vi "RTS APLUS Open Close.vi"(7 "Open Connection?":bool, 8 "error in (no error)":errorcluster, 9 "Modbus Remote Port":u16, 10 "RTS Config Setup Output":T4, 11 "Modbus Connections In":T1={"Wago ModBus Connection"=refnum, "APLUS 1 Modbus Connection"=refnum, "APLUS 2 Modbus Connection"=refnum, "APLUS 3 Modbus Connection"=refnum, "APLUS 4 Modbus Connection"=refnum, "APLUS 5 Modbus Connection"=refnum, "APLUS 6 Modbus Connection"=refnum, "APLUS 7 Modbus Connection"=refnum, "APLUS 8 Modbus Connection"=refnum, "MX 1 VISA Connection"="", "MX 2 VISA Connection"="", "MX 3 VISA Connection"="", "MX 4 VISA Connection"="", "MX 5 VISA Connection"="", "MX1"={"Base Time"=0, "Session Number"=0, "Last Data Number"={"High"=-1, "Low"=4294967295}, "Channel List"=[], "FIFO Number (0)"=0, "Channel Number (1)"=1, "Select FIFO or Channel (F:Channel)"=FALSE, "MX100 Data"={"Measurement Values out"=[], "Date/Time"=""}}, "MX2"={"Base Time"=0, "Session Number"=0, "Last Data Number"={"High"=-1, "Low"=4294967295}, "Channel List"=[], "FIFO Number (0)"=0, "Channel Number (1)"=1, "Select FIFO or Channel (F:Channel)"=FALSE, "MX100 Data"={"Measurement Values out"=[], "Date/Time"=""}}, "MX3"={"Base Time"=0, "Session Number"=0, "Last Data Number"={"High"=-1, "Low"=4294967295}, "Channel List"=[], "FIFO Number (0)"=0, "Channel Number (1)"=1, "Select FIFO or Channel (F:Channel)"=FALSE, "MX100 Data"={"Measurement Values out"=[], "Date/Time"=""}}, "MX4"={"Base Time"=0, "Session Number"=0, "Last Data Number"={"High"=-1, "Low"=4294967295}, "Channel List"=[], "FIFO Number (0)"=0, "Channel Number (1)"=1, "Select FIFO or Channel (F:Channel)"=FALSE, "MX100 Data"={"Measurement Values out"=[], "Date/Time"=""}}, "MX5"={"Base Time"=0, "Session Number"=0, "Last Data Number"={"High"=-1, "Low"=4294967295}, "Channel List"=[], "FIFO Number (0)"=0, "Channel Number (1)"=1, "Select FIFO or Channel (F:Channel)"=FALSE, "MX100 Data"={"Measurement Values out"=[], "Date/Time"=""}}} {"MX5"."Channel Number (1)" min=1 max=60 step=1; "MX5"."FIFO Number (0)" min=-1 max=2 step=1; "MX4"."Channel Number (1)" min=1 max=60 step=1; "MX4"."FIFO Number (0)" min=-1 max=2 step=1; "MX3"."Channel Number (1)" min=1 max=60 step=1; "MX3"."FIFO Number (0)" min=-1 max=2 step=1; "MX2"."Channel Number (1)" min=1 max=60 step=1; "MX2"."FIFO Number (0)" min=-1 max=2 step=1; "MX1"."Channel Number (1)" min=1 max=60 step=1; "MX1"."FIFO Number (0)" min=-1 max=2 step=1}) -> (0 "error out":errorcluster, 3 "Modbus Connections Out":T1={"Wago ModBus Connection"=refnum, "APLUS 1 Modbus Connection"=refnum, "APLUS 2 Modbus Connection"=refnum, "APLUS 3 Modbus Connection"=refnum, "APLUS 4 Modbus Connection"=refnum, "APLUS 5 Modbus Connection"=refnum, "APLUS 6 Modbus Connection"=refnum, "APLUS 7 Modbus Connection"=refnum, "APLUS 8 Modbus Connection"=refnum, "MX 1 VISA Connection"="", "MX 2 VISA Connection"="", "MX 3 VISA Connection"="", "MX 4 VISA Connection"="", "MX 5 VISA Connection"="", "MX1"={"Base Time"=0, "Session Number"=0, "Last Data Number"={"High"=-1, "Low"=4294967295}, "Channel List"=[], "FIFO Number (0)"=0, "Channel Number (1)"=1, "Select FIFO or Channel (F:Channel)"=FALSE, "MX100 Data"={"Measurement Values out"=[], "Date/Time"=""}}, "MX2"={"Base Time"=0, "Session Number"=0, "Last Data Number"={"High"=-1, "Low"=4294967295}, "Channel List"=[], "FIFO Number (0)"=0, "Channel Number (1)"=1, "Select FIFO or Channel (F:Channel)"=FALSE, "MX100 Data"={"Measurement Values out"=[], "Date/Time"=""}}, "MX3"={"Base Time"=0, "Session Number"=0, "Last Data Number"={"High"=-1, "Low"=4294967295}, "Channel List"=[], "FIFO Number (0)"=0, "Channel Number (1)"=1, "Select FIFO or Channel (F:Channel)"=FALSE, "MX100 Data"={"Measurement Values out"=[], "Date/Time"=""}}, "MX4"={"Base Time"=0, "Session Number"=0, "Last Data Number"={"High"=-1, "Low"=4294967295}, "Channel List"=[], "FIFO Number (0)"=0, "Channel Number (1)"=1, "Select FIFO or Channel (F:Channel)"=FALSE, "MX100 Data"={"Measurement Values out"=[], "Date/Time"=""}}, "MX5"={"Base Time"=0, "Session Number"=0, "Last Data Number"={"High"=-1, "Low"=4294967295}, "Channel List"=[], "FIFO Number (0)"=0, "Channel Number (1)"=1, "Select FIFO or Channel (F:Channel)"=FALSE, "MX100 Data"={"Measurement Values out"=[], "Date/Time"=""}}} {"MX5"."Channel Number (1)" min=1 max=60 step=1; "MX5"."FIFO Number (0)" min=-1 max=2 step=1; "MX4"."Channel Number (1)" min=1 max=60 step=1; "MX4"."FIFO Number (0)" min=-1 max=2 step=1; "MX3"."Channel Number (1)" min=1 max=60 step=1; "MX3"."FIFO Number (0)" min=-1 max=2 step=1; "MX2"."Channel Number (1)" min=1 max=60 step=1; "MX2"."FIFO Number (0)" min=-1 max=2 step=1; "MX1"."Channel Number (1)" min=1 max=60 step=1; "MX1"."FIFO Number (0)" min=-1 max=2 step=1})   [LabVIEW 2016]
uses:
  Type Definitions/RTS Modbus Connections.ctl
  <vilib>/NI/Modbus Library/API/Master/Modbus Master.lvclass
  Drivers/Yokogawa MX100/Type Definitions/MX100 Initialization.ctl
  Drivers/Yokogawa MX100/Type Definitions/MX100 Data.ctl
  Type Definitions/RTS Configuration Setup.ctl
  Type Definitions/RTS Wago Config.ctl
  Type Definitions/RTS APLUS Config.ctl
  Type Definitions/RTS Yokogawa MX Config.ctl
  Type Definitions/RTS Replay Server Control.ctl
  Type Definitions/RTS Server Configuration.ctl
  Type Definitions/RTS Station Settions TCP Comms.ctl
  Type Definitions/RTS Chamber Save Status.ctl
  Type Definitions/RTS Test Pattern.ctl
  <vilib>/NI/Modbus Library/API/Wrapper/Create TCP Master.vi
  <vilib>/NI/Modbus Library/API/Wrapper/API Main.lvlib
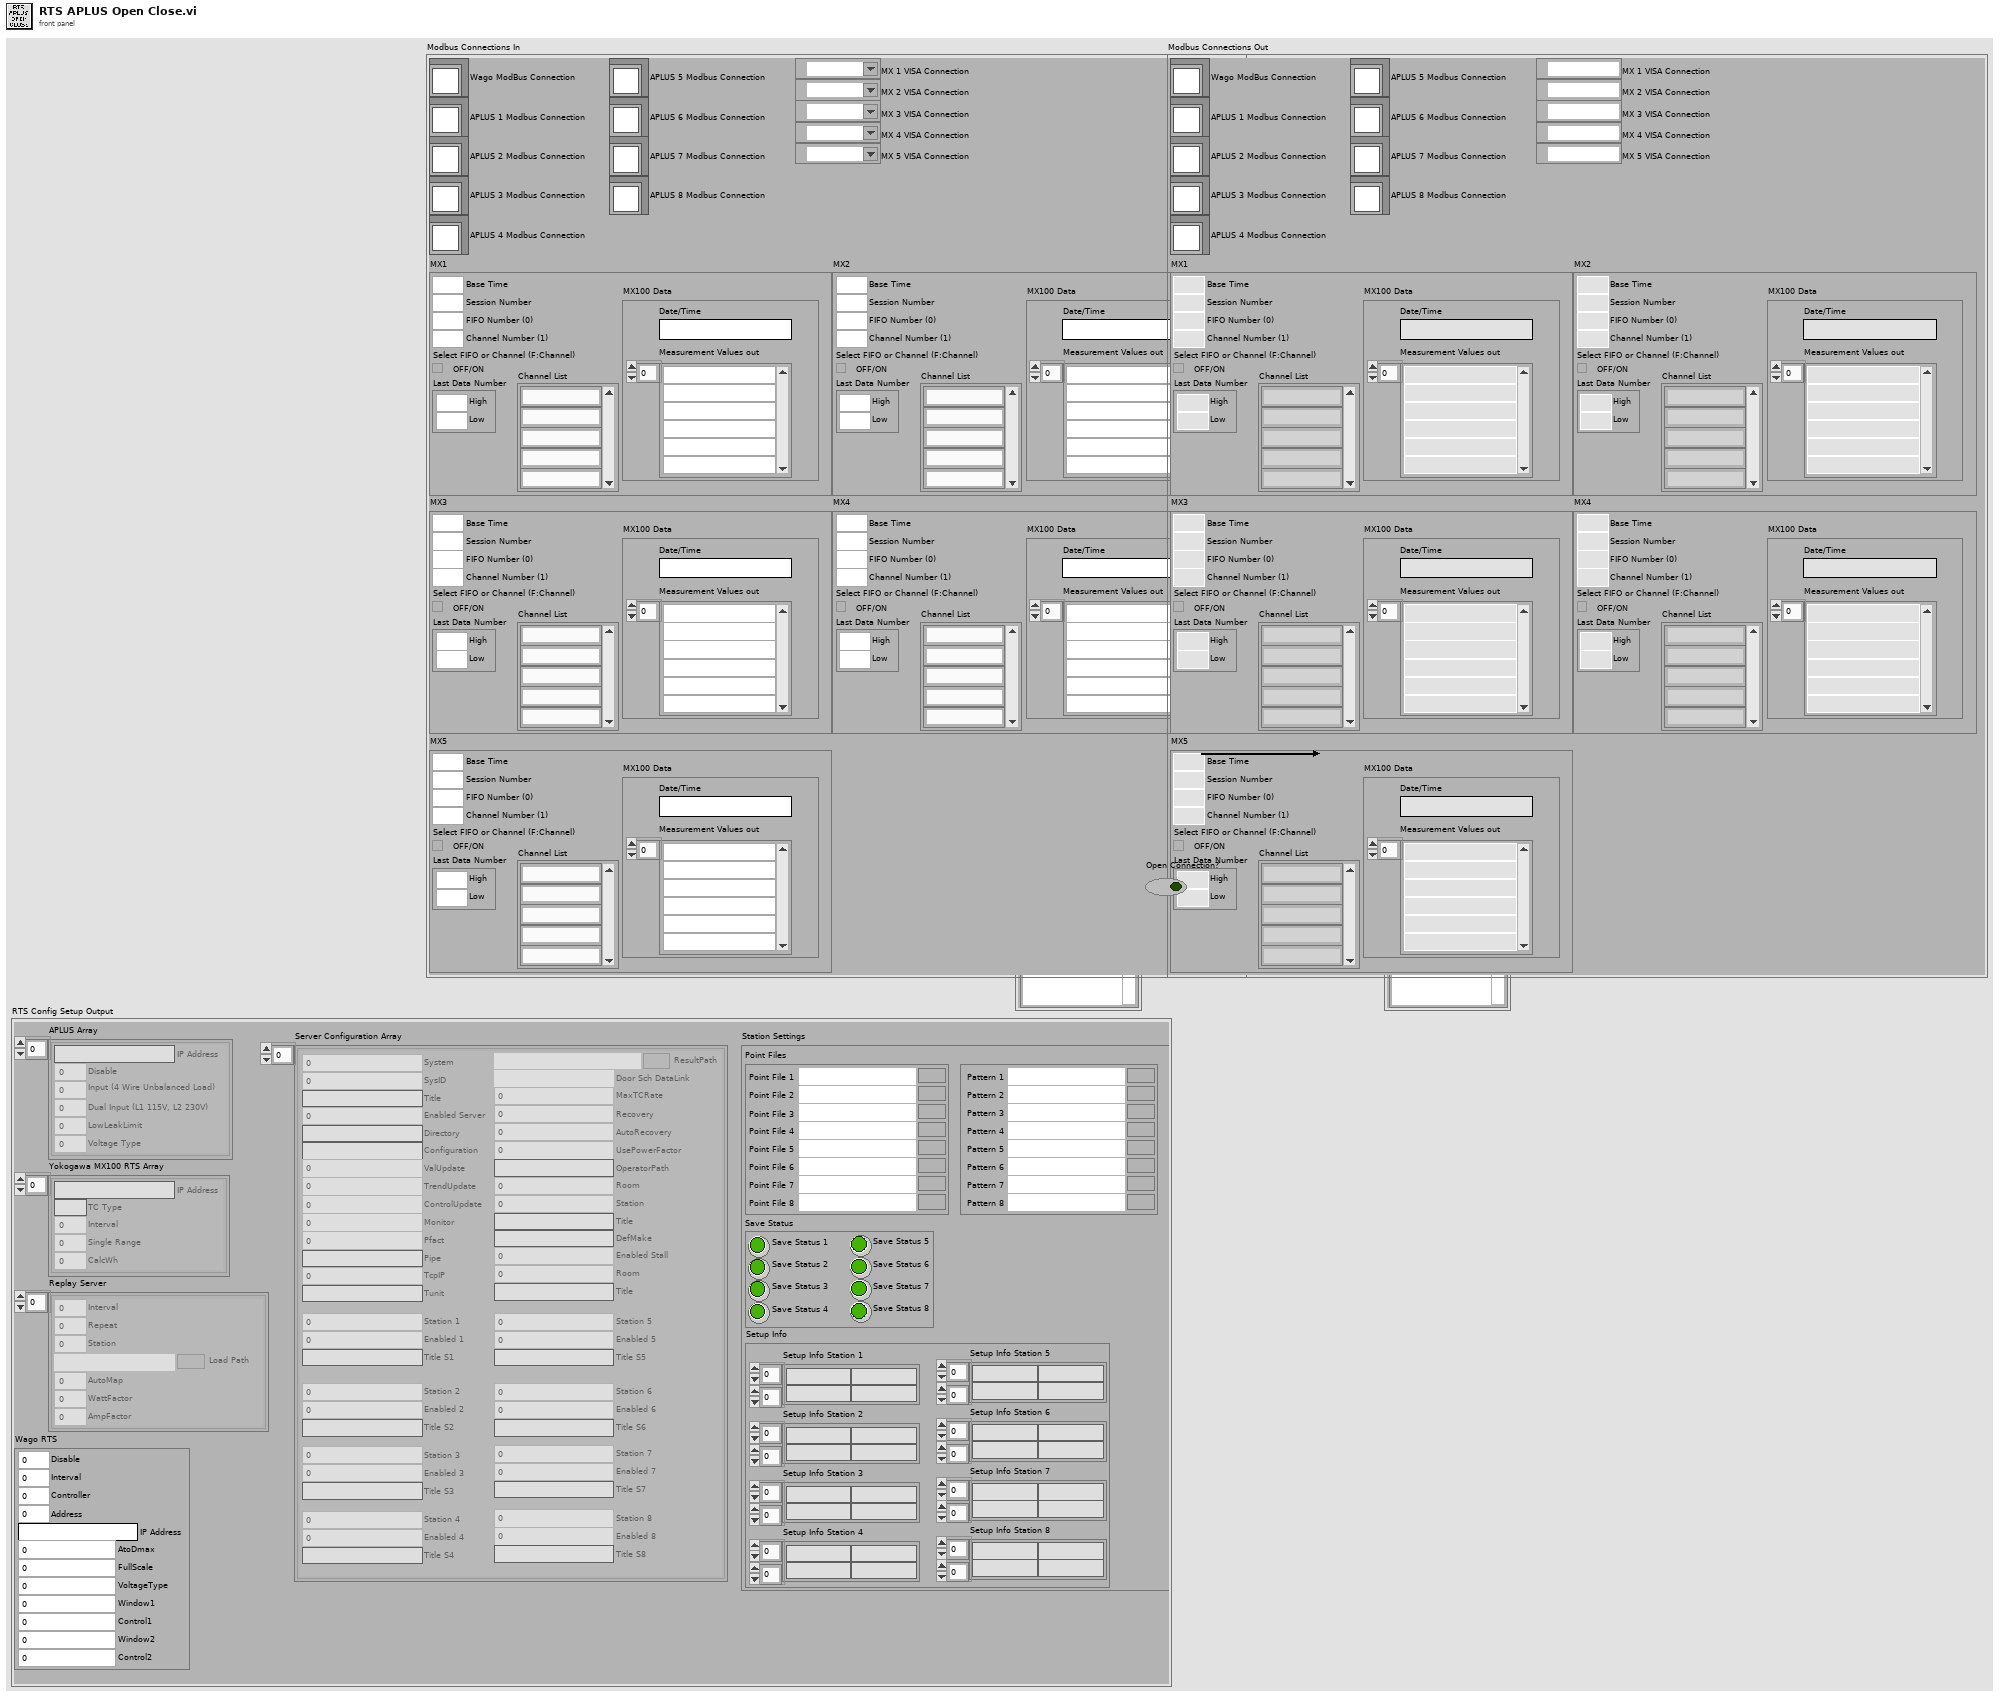
[diagram p1: front panel]
types:
  T1 = typedef "RTS Modbus Connections.ctl" = cluster{"Wago ModBus Connection":refnum<class "Modbus Master.lvclass">, "APLUS 1 Modbus Connection":refnum<class "Modbus Master.lvclass">, "APLUS 2 Modbus Connection":refnum<class "Modbus Master.lvclass">, "APLUS 3 Modbus Connection":refnum<class "Modbus Master.lvclass">, "APLUS 4 Modbus Connection":refnum<class "Modbus Master.lvclass">, "APLUS 5 Modbus Connection":refnum<class "Modbus Master.lvclass">, "APLUS 6 Modbus Connection":refnum<class "Modbus Master.lvclass">, "APLUS 7 Modbus Connection":refnum<class "Modbus Master.lvclass">, "APLUS 8 Modbus Connection":refnum<class "Modbus Master.lvclass">, "MX 1 VISA Connection":refnum<visa-resource-name>, "MX 2 VISA Connection":refnum<visa-resource-name>, "MX 3 VISA Connection":refnum<visa-resource-name>, "MX 4 VISA Connection":refnum<visa-resource-name>, "MX 5 VISA Connection":refnum<visa-resource-name>, "MX1":T2, "MX2":T2, "MX3":T2, "MX4":T2, "MX5":T2}
  T2 = typedef "MX100 Initialization.ctl" = cluster{"Base Time":i32, "Session Number":i32, "Last Data Number":cluster{"High":i32, "Low":u32}, "Channel List":string[], "FIFO Number (0)":i32, "Channel Number (1)":i32, "Select FIFO or Channel (F:Channel)":bool, "MX100 Data":T3}
  T3 = typedef "MX100 Data.ctl" = cluster{"Measurement Values out":dbl[], "Date/Time":string}
  T4 = typedef "RTS Configuration Setup.ctl" = cluster{"Wago RTS":T5, "APLUS Array":T6[], "Yokogawa MX100 RTS Array":T7[], "Replay Server":T8[], "Server Configuration Array":T9[], "Station Settings":T10}
  T5 = typedef "RTS Wago Config.ctl" = cluster{"Disable":u16, "Interval":u16, "Controller":u16, "Address":u16, "IP Address":string, "AtoDmax":u16, "FullScale":u16, "VoltageType":u16, "Window1":u16, "Control1":u16, "Window2":u16, "Control2":u16}
  T6 = typedef "RTS APLUS Config.ctl" = cluster{"Disable":u16, "IP Address":string, "Input (4 Wire Unbalanced Load)":u16, "Dual Input (L1 115V, L2 230V)":u16, "LowLeakLimit":dbl, "Voltage Type":u16}
  T7 = typedef "RTS Yokogawa MX Config.ctl" = cluster{"IP Address":string, "TC Type":string, "Interval":u16, "Single Range":u16, "CalcWh":u16}
  T8 = typedef "RTS Replay Server Control.ctl" = cluster{"Interval":i16, "Repeat":u16, "Station":u16, "Load Path":path, "AutoMap":u16, "WattFactor":dbl, "AmpFactor":dbl}
  T9 = typedef "RTS Server Configuration.ctl" = cluster{"System":u16, "SysID":u16, "Title":string, "Enabled Server":u16, "Directory":string, "Configuration":string, "ValUpdate":u16, "TrendUpdate":u16, "ControlUpdate":u16, "Monitor":u16, "Pfact":u16, "Pipe":string, "TcpIP":u16, "Tunit":string, "ResultPath":path, "Door Sch DataLink":path, "MaxTCRate":u16, "Recovery":u16, "AutoRecovery":u16, "UsePowerFactor":u16, "OperatorPath":string, "Room":u16, "Station":u16, "Title":string, "DefMake":string, "Enabled Stall":u16, "Room":u16, "Title":string, "Station 1":u16, "Enabled 1":u16, "Station 2":u16, "Enabled 2":u16, "Station 3":u16, "Enabled 3":u16, "Station 4":u16, "Enabled 4":u16, "Station 5":u16, "Enabled 5":u16, "Station 6":u16, "Enabled 6":u16, "Station 7":u16, "Enabled 7":u16, "Station 8":u16, "Enabled 8":u16, "Title S1":string, "Title S2":string, "Title S3":string, "Title S5":string, "Title S6":string, "Title S7":string, "Title S8":string, "Title S4":string}
  T10 = typedef "RTS Station Settions TCP Comms.ctl" = cluster{"Point Files":cluster{"Point File 1":path, "Point File 2":path, "Point File 3":path, "Point File 4":path, "Point File 5":path, "Point File 6":path, "Point File 7":path, "Point File 8":path}, "Save Status":T11, "Setup Info":cluster{"Setup Info Station 1":string[][], "Setup Info Station 2":string[][], "Setup Info Station 3":string[][], "Setup Info Station 4":string[][], "Setup Info Station 5":string[][], "Setup Info Station 6":string[][], "Setup Info Station 7":string[][], "Setup Info Station 8":string[][]}, "Chamber Test Pattern":T12}
  T11 = typedef "RTS Chamber Save Status.ctl" = cluster{"Save Status 1":bool, "Save Status 2":bool, "Save Status 3":bool, "Save Status 4":bool, "Save Status 5":bool, "Save Status 6":bool, "Save Status 7":bool, "Save Status 8":bool}
  T12 = typedef "RTS Test Pattern.ctl" = cluster{" Pattern 1":path, "Pattern 2":path, "Pattern 3":path, "Pattern 4":path, "Pattern 5":path, "Pattern 6":path, "Pattern 7":path, "Pattern 8":path}
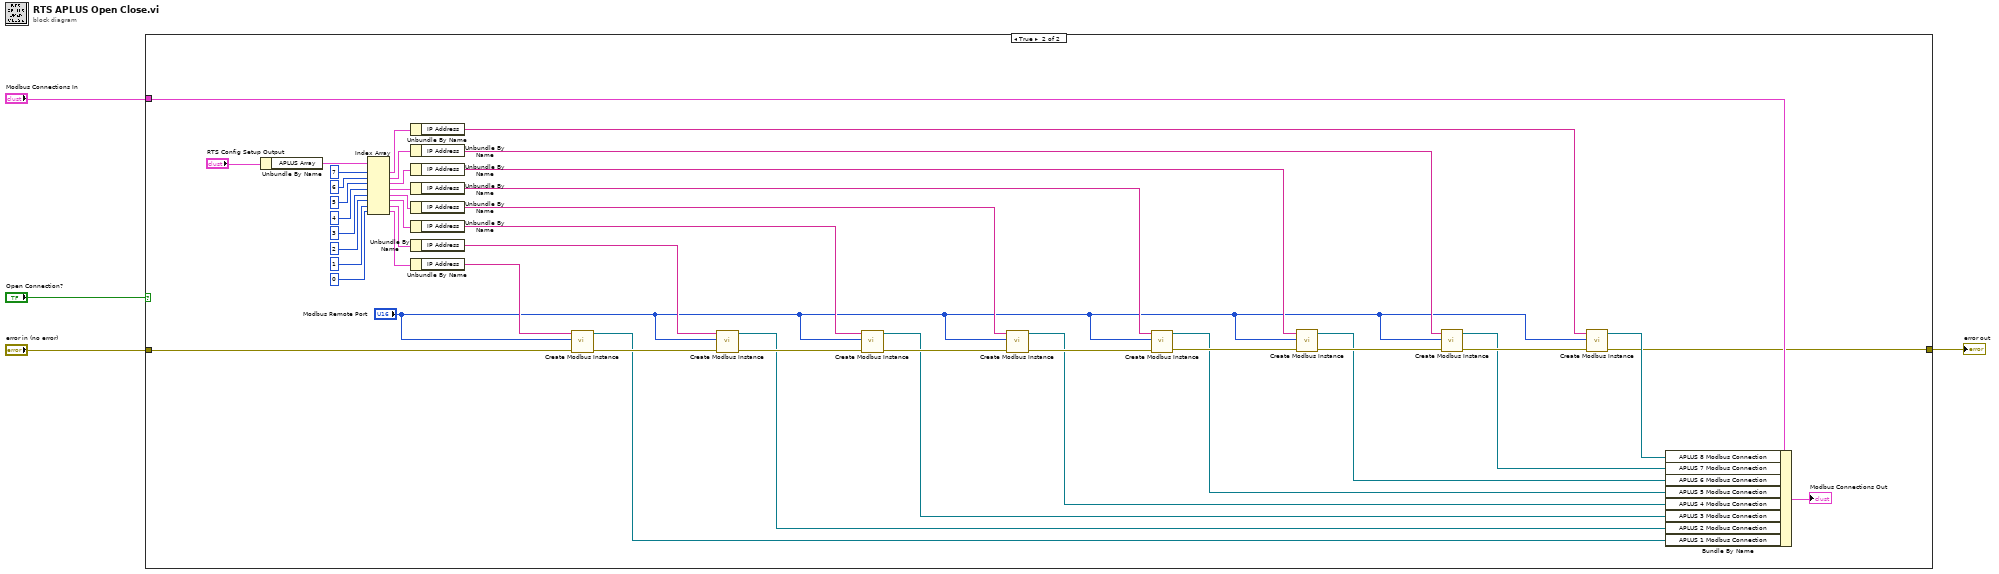
[diagram p0: block diagram]
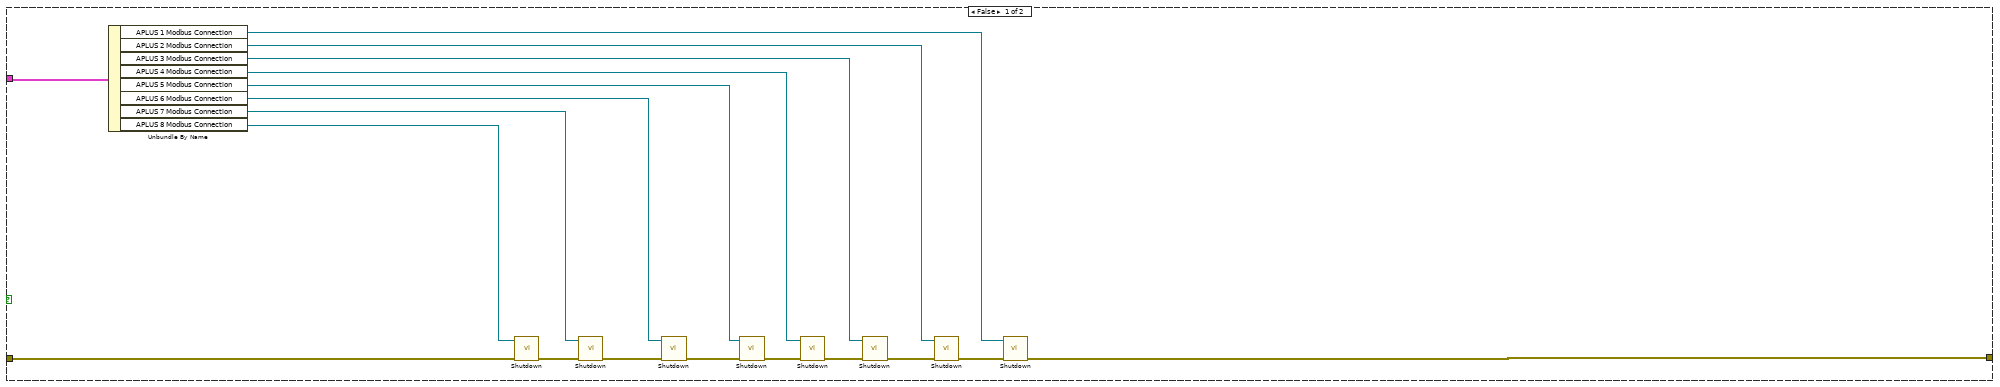
[diagram p2: hidden frame]
diagram:
  n1 = case shown="True" "Open Connection?" {
    tunnel: "Modbus Connections In" -> [w22 w64]
    tunnel: "error in (no error)" -> [w21 w25]
    tunnel: [w13 w24] -> w1
    frame False {
      n2 = Unbundle By Name(w22) -> ("APLUS 1 Modbus Connection"=w5:refnum<class "Modbus Master.lvclass">, "APLUS 2 Modbus Connection"=w6:refnum<class "Modbus Master.lvclass">, "APLUS 3 Modbus Connection"=w7:refnum<class "Modbus Master.lvclass">, "APLUS 4 Modbus Connection"=w8:refnum<class "Modbus Master.lvclass">, "APLUS 5 Modbus Connection"=w9:refnum<class "Modbus Master.lvclass">, "APLUS 6 Modbus Connection"=w10:refnum<class "Modbus Master.lvclass">, "APLUS 7 Modbus Connection"=w11:refnum<class "Modbus Master.lvclass">, "APLUS 8 Modbus Connection"=w12:refnum<class "Modbus Master.lvclass">)
      n3 = call-dynamic "Shutdown.vi"("error in"=w21, "Modbus master in"=w12) -> ("error out"=w20:errorcluster)  [unwired: 9 in]
      n4 = call-dynamic "Shutdown.vi"("error in"=w20, "Modbus master in"=w11) -> ("error out"=w19:errorcluster)  [unwired: 9 in]
      n5 = call-dynamic "Shutdown.vi"("error in"=w19, "Modbus master in"=w10) -> ("error out"=w18:errorcluster)  [unwired: 9 in]
      n6 = call-dynamic "Shutdown.vi"("error in"=w18, "Modbus master in"=w9) -> ("error out"=w17:errorcluster)  [unwired: 9 in]
      n7 = call-dynamic "Shutdown.vi"("error in"=w17, "Modbus master in"=w8) -> ("error out"=w16:errorcluster)  [unwired: 9 in]
      n8 = call-dynamic "Shutdown.vi"("error in"=w16, "Modbus master in"=w7) -> ("error out"=w15:errorcluster)  [unwired: 9 in]
      n9 = call-dynamic "Shutdown.vi"("error in"=w15, "Modbus master in"=w6) -> ("error out"=w14:errorcluster)  [unwired: 9 in]
      n10 = call-dynamic "Shutdown.vi"("error in"=w14, "Modbus master in"=w5) -> ("error out"=w13:errorcluster)  [unwired: 9 in]
    }
    frame True {
      n11 = Unbundle By Name("RTS Config Setup Output") -> ("APLUS Array"=w65:T6[])
      n12 = Index Array(array=w65, index #1=7 ("index"), index #2=6 ("index"), index #3=5 ("index"), index #4=4 ("index"), index #5=3 ("index"), index #6=2 ("index"), index #7=1 ("index"), index #8=0 ("index")) -> (element #1=w48:T6, element #2=w49:T6, element #3=w50:T6, element #4=w51:T6, element #5=w52:T6, element #6=w53:T6, element #7=w54:T6, element #8=w55:T6)
      n13 = Unbundle By Name(w48) -> ("IP Address"=w41:string)
      n14 = Unbundle By Name(w49) -> ("IP Address"=w42:string)
      n15 = Unbundle By Name(w50) -> ("IP Address"=w43:string)
      n16 = Unbundle By Name(w51) -> ("IP Address"=w44:string)
      n17 = Unbundle By Name(w52) -> ("IP Address"=w45:string)
      n18 = Unbundle By Name(w53) -> ("IP Address"=w46:string)
      n19 = Unbundle By Name(w54) -> ("IP Address"=w47:string)
      n20 = Unbundle By Name(w55) -> ("IP Address"=w68:string)
      n21 = call-poly <vilib>:"Create Modbus Instance.vi"("error in"=w25, "port (502)"="Modbus Remote Port", "address"=w68) -> ("error out"=w34:errorcluster, "TCP master instance"=w33:refnum<class "Modbus Master.lvclass">)  [unwired: 7 in]
      n22 = call-poly <vilib>:"Create Modbus Instance.vi"("error in"=w34, "port (502)"="Modbus Remote Port", "address"=w47) -> ("error out"=w35:errorcluster, "TCP master instance"=w32:refnum<class "Modbus Master.lvclass">)  [unwired: 7 in]
      n23 = call-poly <vilib>:"Create Modbus Instance.vi"("error in"=w35, "port (502)"="Modbus Remote Port", "address"=w46) -> ("error out"=w36:errorcluster, "TCP master instance"=w31:refnum<class "Modbus Master.lvclass">)  [unwired: 7 in]
      n24 = call-poly <vilib>:"Create Modbus Instance.vi"("error in"=w36, "port (502)"="Modbus Remote Port", "address"=w45) -> ("error out"=w37:errorcluster, "TCP master instance"=w30:refnum<class "Modbus Master.lvclass">)  [unwired: 7 in]
      n25 = call-poly <vilib>:"Create Modbus Instance.vi"("error in"=w37, "port (502)"="Modbus Remote Port", "address"=w44) -> ("error out"=w38:errorcluster, "TCP master instance"=w29:refnum<class "Modbus Master.lvclass">)  [unwired: 7 in]
      n26 = call-poly <vilib>:"Create Modbus Instance.vi"("error in"=w38, "port (502)"="Modbus Remote Port", "address"=w43) -> ("error out"=w39:errorcluster, "TCP master instance"=w28:refnum<class "Modbus Master.lvclass">)  [unwired: 7 in]
      n27 = call-poly <vilib>:"Create Modbus Instance.vi"("error in"=w39, "port (502)"="Modbus Remote Port", "address"=w42) -> ("error out"=w40:errorcluster, "TCP master instance"=w27:refnum<class "Modbus Master.lvclass">)  [unwired: 7 in]
      n28 = call-poly <vilib>:"Create Modbus Instance.vi"("error in"=w40, "port (502)"="Modbus Remote Port", "address"=w41) -> ("error out"=w24:errorcluster, "TCP master instance"=w26:refnum<class "Modbus Master.lvclass">)  [unwired: 7 in]
      n29 = Bundle By Name(cluster=w64, "APLUS 8 Modbus Connection"=w26, "APLUS 7 Modbus Connection"=w27, "APLUS 6 Modbus Connection"=w28, "APLUS 5 Modbus Connection"=w29, "APLUS 4 Modbus Connection"=w30, "APLUS 3 Modbus Connection"=w31, "APLUS 2 Modbus Connection"=w32, "APLUS 1 Modbus Connection"=w33) -> (→"Modbus Connections Out":T1)
    }
  }
  "error out" <- w1
